vi "Set Up Dialog - Force.vi"() -> ()   [LabVIEW 2012]
panel:
  out "Calibration Instructions":string="1. Connect the sensor to your myDAQ as shown in the diagram above.\n\n2. Select the force range you would like to use (500g or 5Kg).\n\n3. Start with no load on the FTN-5k and record the voltage SP2 Voltage (0 kgf). This will 'tare' the device for no load.\n\n4. Hang a known mass from the FTN-5k, enter the value of the mass in SP1 Value, then record the voltage for SP2."
  # "iWorx - Force - Set Up"
  # "Force Sensor (FTN - 5k)"
  # "iWorx"
  # "Computer"
  # "Sensor"
  # "FTN - 5k"
  # "myDAQ"
  # "Adaptor"
  # "Connection Diagram"
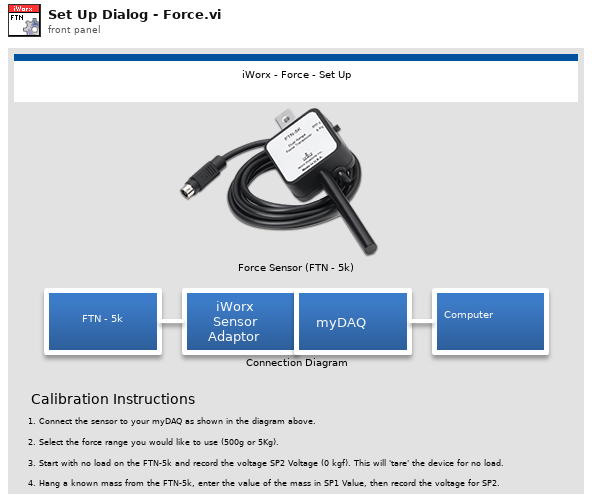
[diagram p1: front panel]
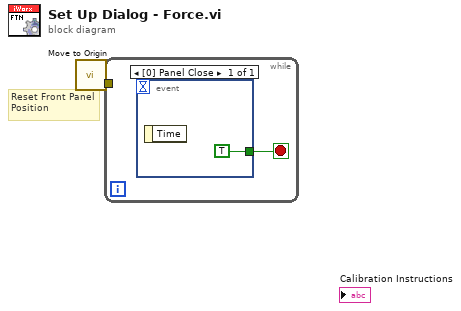
[diagram p0: block diagram]
diagram:
  # "Reset Front Panel Position"
  n1 = call "Move to Origin.vi"() -> ("Error Out"=w1:errorcluster)  [unwired: 3 in]
  n2 = while {
    tunnel: w1 -> [_]
    stop <- w2 stop-if-true
    n3 = event shown="[0] Panel Close" {
      selector: _ -> [_]
      dyn-events: _ -> [_]
      timeout: _ -> [_]
      tunnel: [TRUE] -> w2
      event Panel Close {
        n4 = event-data() -> ()  [unwired: 1 in, 1 out]
      }
    }
  }
